vi "PicoScopeospaExampleAdvancedTrigger.vi"() -> ()   [LabVIEW 2010]
uses:
  shared/PicoBuffers.ctl
  <vilib>/Waveform/DWDTOps.llb/DWDT Analog to Digital.vi
  PicoScopepsospaLib/PicoScopeospaDigitalChannelSettings.ctl
  shared/Acquisition Settings.ctl
  shared/Buffer and Transfer Settings.ctl
  PicoScopepsospaLib/PicoScopeospaAnalogChannelSettings.ctl
panel:
  in  "Write ChA to file":bool
  in  "Channels":T1={"Channel A Settings "={"Enabled"=TRUE, "Coupling"=1, "Range"=8, "Analogue Offset"=0.0, "BandWidth"=0, "PROBE_RANGE_INFO"=0}, "Channel B Settings "={"Enabled"=FALSE, "Coupling"=1, "Range"=8, "Analogue Offset"=0.0, "BandWidth"=0, "PROBE_RANGE_INFO"=0}, "Channel C Settings "={"Enabled"=FALSE, "Coupling"=1, "Range"=8, "Analogue Offset"=0.0, "BandWidth"=0, "PROBE_RANGE_INFO"=0}, "Channel D Settings "={"Enabled"=FALSE, "Coupling"=1, "Range"=8, "Analogue Offset"=0.0, "BandWidth"=0, "PROBE_RANGE_INFO"=0}, "Channel E Settings "={"Enabled"=FALSE, "Coupling"=1, "Range"=8, "Analogue Offset"=0.0, "BandWidth"=0, "PROBE_RANGE_INFO"=0}, "Channel F Settings "={"Enabled"=FALSE, "Coupling"=1, "Range"=8, "Analogue Offset"=0.0, "BandWidth"=0, "PROBE_RANGE_INFO"=0}, "Channel G Settings "={"Enabled"=FALSE, "Coupling"=1, "Range"=8, "Analogue Offset"=0.0, "BandWidth"=0, "PROBE_RANGE_INFO"=0}, "Channel H Settings "={"Enabled"=FALSE, "Coupling"=1, "Range"=8, "Analogue Offset"=0.0, "BandWidth"=0, "PROBE_RANGE_INFO"=0}} {"Channel H Settings"."PROBE_RANGE_INFO" items=["PROBE_NONE_NV"=0, "X1_PROBE_NV"=1, "X10_PROBE_NV"=10]; "Channel H Settings"."BandWidth" items=["Full"=0, "100kHz"=100000, "20kHz"=200000, "1MHz"=1000000, "20MHz"=20000000, "25MHz"=25000000, "50MHz"=50000000, "200MHz"=200000000, "250MHz"=250000000, "500MHz"=500000000]; "Channel H Settings"."Range" items=["10mV"=0, "20mV"=1, "50mV"=2, "100mV"=3, "200mV"=4, "500mV"=5, "1V"=6, "2V"=7, "5V"=8, "10V"=9, "20V"=10, "50V"=11, "100V"=12, "200V"=13, "x10_Probe_100mV"=32, "x10_Probe_200mV"=33, "x10_Probe_500mV"=34, "x10_Probe_1V"=35, "x10_Probe_2V"=36, "x10_Probe_5V"=37, "x10_Probe_10V"=38, "x10_Probe_20V"=39, "x10_Probe_50V"=40, "x10_Probe_100V"=41, "x10_Probe_200V"=42, "x10_Probe_500V"=43, "CURRENT_CLAMP_60A_2A"=10500, "CURRENT_CLAMP_60A_5A"=10501, "CURRENT_CLAMP_60A_10A"=10502, "CURRENT_CLAMP_60A_20A"=10503, "CURRENT_CLAMP_60A_50A"=10504, "CURRENT_CLAMP_60A_60A"=10505, "CURRENT_CLAMP_60A_V2_0_5A"=10600, "CURRENT_CLAMP_60A_V2_1A"=10601, "CURRENT_CLAMP_60A_V2_2A"=10602, "CURRENT_CLAMP_60A_V2_5A"=10603, "CURRENT_CLAMP_60A_V2_10A"=10604, "CURRENT_CLAMP_60A_V2_20A"=10605, "CURRENT_CLAMP_60A_V2_50A"=10606, "CURRENT_CLAMP_60A_V2_60A"=10607, "RESISTANCE_LEAD_NEG5_TO_20OHM"=7000, "RESISTANCE_LEAD_NEG50_TO_200OHM"=7001, "RESISTANCE_LEAD_NEG500_TO_2KOHM"=7002, "RESISTANCE_LEAD_NEG5K_TO_20KOHM"=7003, "RESISTANCE_LEAD_NEG50K_TO_LEAD_200KOHM"=7004, "RESISTANCE_LEAD_NEG500K_TO_LEAD_2MOHM"=7005, "RESISTANCE_LEAD_DIODE_TEST"=7006, "HT_NEG3_TO_5KV"=8950, "HT_NEG3_TO_10KV"=8951, "HT_NEG5_TO_20KV"=8952, "HT_NEG5_TO_50KV"=8953, "HT_NEG5_TO_100KV"=8954, "HT_NEG3_TO_5KV_INVERTED"=8955, "HT_NEG3_TO_10KV_INVERTED"=8956, "HT_NEG5_TO_20KV_INVERTED"=8957, "HT_NEG5_TO_50KV_INVERTED"=8958, "HT_NEG5_TO_100KV_INVERTED"=8959, "TEMPERATURE_NEG50_TO_150DEGC"=9000, "PRESSURE_SENSOR_-100k-150k_PASCALS"=9100, "PRESSURE_SENSOR_-100k_TO_400k_PASCALS"=9101, "PRESSURE_SENSOR_-200k_TO_800k_PASCALS"=9102, "PRESSURE_SENSOR_-400k_TO_1600k_PASCALS"=9103, "PRESSURE_SENSOR_-400k_TO_3400k_PASCALS"=9104, "PRESSURE_SENSOR_-150k_TO_1350k_PASCALS"=9105]; "Channel H Settings"."Coupling" items=["AC"=0, "DC 1M Ohm"=1, "DC 50 Ohm"=50]; "Channel G Settings"."PROBE_RANGE_INFO" items=["PROBE_NONE_NV"=0, "X1_PROBE_NV"=1, "X10_PROBE_NV"=10]; "Channel G Settings"."BandWidth" items=["Full"=0, "100kHz"=100000, "20kHz"=200000, "1MHz"=1000000, "20MHz"=20000000, "25MHz"=25000000, "50MHz"=50000000, "200MHz"=200000000, "250MHz"=250000000, "500MHz"=500000000]; "Channel G Settings"."Range" items=["10mV"=0, "20mV"=1, "50mV"=2, "100mV"=3, "200mV"=4, "500mV"=5, "1V"=6, "2V"=7, "5V"=8, "10V"=9, "20V"=10, "50V"=11, "100V"=12, "200V"=13, "x10_Probe_100mV"=32, "x10_Probe_200mV"=33, "x10_Probe_500mV"=34, "x10_Probe_1V"=35, "x10_Probe_2V"=36, "x10_Probe_5V"=37, "x10_Probe_10V"=38, "x10_Probe_20V"=39, "x10_Probe_50V"=40, "x10_Probe_100V"=41, "x10_Probe_200V"=42, "x10_Probe_500V"=43, "CURRENT_CLAMP_60A_2A"=10500, "CURRENT_CLAMP_60A_5A"=10501, "CURRENT_CLAMP_60A_10A"=10502, "CURRENT_CLAMP_60A_20A"=10503, "CURRENT_CLAMP_60A_50A"=10504, "CURRENT_CLAMP_60A_60A"=10505, "CURRENT_CLAMP_60A_V2_0_5A"=10600, "CURRENT_CLAMP_60A_V2_1A"=10601, "CURRENT_CLAMP_60A_V2_2A"=10602, "CURRENT_CLAMP_60A_V2_5A"=10603, "CURRENT_CLAMP_60A_V2_10A"=10604, "CURRENT_CLAMP_60A_V2_20A"=10605, "CURRENT_CLAMP_60A_V2_50A"=10606, "CURRENT_CLAMP_60A_V2_60A"=10607, "RESISTANCE_LEAD_NEG5_TO_20OHM"=7000, "RESISTANCE_LEAD_NEG50_TO_200OHM"=7001, "RESISTANCE_LEAD_NEG500_TO_2KOHM"=7002, "RESISTANCE_LEAD_NEG5K_TO_20KOHM"=7003, "RESISTANCE_LEAD_NEG50K_TO_LEAD_200KOHM"=7004, "RESISTANCE_LEAD_NEG500K_TO_LEAD_2MOHM"=7005, "RESISTANCE_LEAD_DIODE_TEST"=7006, "HT_NEG3_TO_5KV"=8950, "HT_NEG3_TO_10KV"=8951, "HT_NEG5_TO_20KV"=8952, "HT_NEG5_TO_50KV"=8953, "HT_NEG5_TO_100KV"=8954, "HT_NEG3_TO_5KV_INVERTED"=8955, "HT_NEG3_TO_10KV_INVERTED"=8956, "HT_NEG5_TO_20KV_INVERTED"=8957, "HT_NEG5_TO_50KV_INVERTED"=8958, "HT_NEG5_TO_100KV_INVERTED"=8959, "TEMPERATURE_NEG50_TO_150DEGC"=9000, "PRESSURE_SENSOR_-100k-150k_PASCALS"=9100, "PRESSURE_SENSOR_-100k_TO_400k_PASCALS"=9101, "PRESSURE_SENSOR_-200k_TO_800k_PASCALS"=9102, "PRESSURE_SENSOR_-400k_TO_1600k_PASCALS"=9103, "PRESSURE_SENSOR_-400k_TO_3400k_PASCALS"=9104, "PRESSURE_SENSOR_-150k_TO_1350k_PASCALS"=9105]; "Channel G Settings"."Coupling" items=["AC"=0, "DC 1M Ohm"=1, "DC 50 Ohm"=50]; "Channel F Settings"."PROBE_RANGE_INFO" items=["PROBE_NONE_NV"=0, "X1_PROBE_NV"=1, "X10_PROBE_NV"=10]; "Channel F Settings"."BandWidth" items=["Full"=0, "100kHz"=100000, "20kHz"=200000, "1MHz"=1000000, "20MHz"=20000000, "25MHz"=25000000, "50MHz"=50000000, "200MHz"=200000000, "250MHz"=250000000, "500MHz"=500000000]; "Channel F Settings"."Range" items=["10mV"=0, "20mV"=1, "50mV"=2, "100mV"=3, "200mV"=4, "500mV"=5, "1V"=6, "2V"=7, "5V"=8, "10V"=9, "20V"=10, "50V"=11, "100V"=12, "200V"=13, "x10_Probe_100mV"=32, "x10_Probe_200mV"=33, "x10_Probe_500mV"=34, "x10_Probe_1V"=35, "x10_Probe_2V"=36, "x10_Probe_5V"=37, "x10_Probe_10V"=38, "x10_Probe_20V"=39, "x10_Probe_50V"=40, "x10_Probe_100V"=41, "x10_Probe_200V"=42, "x10_Probe_500V"=43, "CURRENT_CLAMP_60A_2A"=10500, "CURRENT_CLAMP_60A_5A"=10501, "CURRENT_CLAMP_60A_10A"=10502, "CURRENT_CLAMP_60A_20A"=10503, "CURRENT_CLAMP_60A_50A"=10504, "CURRENT_CLAMP_60A_60A"=10505, "CURRENT_CLAMP_60A_V2_0_5A"=10600, "CURRENT_CLAMP_60A_V2_1A"=10601, "CURRENT_CLAMP_60A_V2_2A"=10602, "CURRENT_CLAMP_60A_V2_5A"=10603, "CURRENT_CLAMP_60A_V2_10A"=10604, "CURRENT_CLAMP_60A_V2_20A"=10605, "CURRENT_CLAMP_60A_V2_50A"=10606, "CURRENT_CLAMP_60A_V2_60A"=10607, "RESISTANCE_LEAD_NEG5_TO_20OHM"=7000, "RESISTANCE_LEAD_NEG50_TO_200OHM"=7001, "RESISTANCE_LEAD_NEG500_TO_2KOHM"=7002, "RESISTANCE_LEAD_NEG5K_TO_20KOHM"=7003, "RESISTANCE_LEAD_NEG50K_TO_LEAD_200KOHM"=7004, "RESISTANCE_LEAD_NEG500K_TO_LEAD_2MOHM"=7005, "RESISTANCE_LEAD_DIODE_TEST"=7006, "HT_NEG3_TO_5KV"=8950, "HT_NEG3_TO_10KV"=8951, "HT_NEG5_TO_20KV"=8952, "HT_NEG5_TO_50KV"=8953, "HT_NEG5_TO_100KV"=8954, "HT_NEG3_TO_5KV_INVERTED"=8955, "HT_NEG3_TO_10KV_INVERTED"=8956, "HT_NEG5_TO_20KV_INVERTED"=8957, "HT_NEG5_TO_50KV_INVERTED"=8958, "HT_NEG5_TO_100KV_INVERTED"=8959, "TEMPERATURE_NEG50_TO_150DEGC"=9000, "PRESSURE_SENSOR_-100k-150k_PASCALS"=9100, "PRESSURE_SENSOR_-100k_TO_400k_PASCALS"=9101, "PRESSURE_SENSOR_-200k_TO_800k_PASCALS"=9102, "PRESSURE_SENSOR_-400k_TO_1600k_PASCALS"=9103, "PRESSURE_SENSOR_-400k_TO_3400k_PASCALS"=9104, "PRESSURE_SENSOR_-150k_TO_1350k_PASCALS"=9105]; "Channel F Settings"."Coupling" items=["AC"=0, "DC 1M Ohm"=1, "DC 50 Ohm"=50]; "Channel E Settings"."PROBE_RANGE_INFO" items=["PROBE_NONE_NV"=0, "X1_PROBE_NV"=1, "X10_PROBE_NV"=10]; "Channel E Settings"."BandWidth" items=["Full"=0, "100kHz"=100000, "20kHz"=200000, "1MHz"=1000000, "20MHz"=20000000, "25MHz"=25000000, "50MHz"=50000000, "200MHz"=200000000, "250MHz"=250000000, "500MHz"=500000000]; "Channel E Settings"."Range" items=["10mV"=0, "20mV"=1, "50mV"=2, "100mV"=3, "200mV"=4, "500mV"=5, "1V"=6, "2V"=7, "5V"=8, "10V"=9, "20V"=10, "50V"=11, "100V"=12, "200V"=13, "x10_Probe_100mV"=32, "x10_Probe_200mV"=33, "x10_Probe_500mV"=34, "x10_Probe_1V"=35, "x10_Probe_2V"=36, "x10_Probe_5V"=37, "x10_Probe_10V"=38, "x10_Probe_20V"=39, "x10_Probe_50V"=40, "x10_Probe_100V"=41, "x10_Probe_200V"=42, "x10_Probe_500V"=43, "CURRENT_CLAMP_60A_2A"=10500, "CURRENT_CLAMP_60A_5A"=10501, "CURRENT_CLAMP_60A_10A"=10502, "CURRENT_CLAMP_60A_20A"=10503, "CURRENT_CLAMP_60A_50A"=10504, "CURRENT_CLAMP_60A_60A"=10505, "CURRENT_CLAMP_60A_V2_0_5A"=10600, "CURRENT_CLAMP_60A_V2_1A"=10601, "CURRENT_CLAMP_60A_V2_2A"=10602, "CURRENT_CLAMP_60A_V2_5A"=10603, "CURRENT_CLAMP_60A_V2_10A"=10604, "CURRENT_CLAMP_60A_V2_20A"=10605, "CURRENT_CLAMP_60A_V2_50A"=10606, "CURRENT_CLAMP_60A_V2_60A"=10607, "RESISTANCE_LEAD_NEG5_TO_20OHM"=7000, "RESISTANCE_LEAD_NEG50_TO_200OHM"=7001, "RESISTANCE_LEAD_NEG500_TO_2KOHM"=7002, "RESISTANCE_LEAD_NEG5K_TO_20KOHM"=7003, "RESISTANCE_LEAD_NEG50K_TO_LEAD_200KOHM"=7004, "RESISTANCE_LEAD_NEG500K_TO_LEAD_2MOHM"=7005, "RESISTANCE_LEAD_DIODE_TEST"=7006, "HT_NEG3_TO_5KV"=8950, "HT_NEG3_TO_10KV"=8951, "HT_NEG5_TO_20KV"=8952, "HT_NEG5_TO_50KV"=8953, "HT_NEG5_TO_100KV"=8954, "HT_NEG3_TO_5KV_INVERTED"=8955, "HT_NEG3_TO_10KV_INVERTED"=8956, "HT_NEG5_TO_20KV_INVERTED"=8957, "HT_NEG5_TO_50KV_INVERTED"=8958, "HT_NEG5_TO_100KV_INVERTED"=8959, "TEMPERATURE_NEG50_TO_150DEGC"=9000, "PRESSURE_SENSOR_-100k-150k_PASCALS"=9100, "PRESSURE_SENSOR_-100k_TO_400k_PASCALS"=9101, "PRESSURE_SENSOR_-200k_TO_800k_PASCALS"=9102, "PRESSURE_SENSOR_-400k_TO_1600k_PASCALS"=9103, "PRESSURE_SENSOR_-400k_TO_3400k_PASCALS"=9104, "PRESSURE_SENSOR_-150k_TO_1350k_PASCALS"=9105]; "Channel E Settings"."Coupling" items=["AC"=0, "DC 1M Ohm"=1, "DC 50 Ohm"=50]; "Channel D Settings"."BandWidth" items=["Full"=0, "100kHz"=100000, "20kHz"=200000, "1MHz"=1000000, "20MHz"=20000000, "25MHz"=25000000, "50MHz"=50000000, "100MHz"=100000000, "200MHz"=200000000, "250MHz"=250000000, "350MHz"=350000000, "500MHz"=500000000]; "Channel D Settings"."PROBE_RANGE_INFO" items=["PROBE_NONE_NV"=0, "X1_PROBE_NV"=1, "X10_PROBE_NV"=10]; "Channel D Settings"."Range" items=["10mV", "20mV", "50mV", "100mV", "200mV", "500mV", "1V", "2V", "5V", "10V", "20V", "50V", "100V", "200V"]; "Channel D Settings"."Coupling" items=["AC"=0, "DC 1M Ohm"=1, "DC 50 Ohm"=50]; "Channel C Settings"."BandWidth" items=["Full"=0, "100kHz"=100000, "20kHz"=200000, "1MHz"=1000000, "20MHz"=20000000, "25MHz"=25000000, "50MHz"=50000000, "100MHz"=100000000, "200MHz"=200000000, "250MHz"=250000000, "350MHz"=350000000, "500MHz"=500000000]; "Channel C Settings"."PROBE_RANGE_INFO" items=["PROBE_NONE_NV"=0, "X1_PROBE_NV"=1, "X10_PROBE_NV"=10]; "Channel C Settings"."Range" items=["10mV", "20mV", "50mV", "100mV", "200mV", "500mV", "1V", "2V", "5V", "10V", "20V", "50V", "100V", "200V"]; "Channel C Settings"."Coupling" items=["AC"=0, "DC 1M Ohm"=1, "DC 50 Ohm"=50]; "Channel B Settings"."BandWidth" items=["Full"=0, "100kHz"=100000, "20kHz"=200000, "1MHz"=1000000, "20MHz"=20000000, "25MHz"=25000000, "50MHz"=50000000, "100MHz"=100000000, "200MHz"=200000000, "250MHz"=250000000, "350MHz"=350000000, "500MHz"=500000000]; "Channel B Settings"."PROBE_RANGE_INFO" items=["PROBE_NONE_NV"=0, "X1_PROBE_NV"=1, "X10_PROBE_NV"=10]; "Channel B Settings"."Range" items=["10mV", "20mV", "50mV", "100mV", "200mV", "500mV", "1V", "2V", "5V", "10V", "20V", "50V", "100V", "200V"]; "Channel B Settings"."Coupling" items=["AC"=0, "DC 1M Ohm"=1, "DC 50 Ohm"=50]; "Channel A Settings"."PROBE_RANGE_INFO" items=["PROBE_NONE_NV"=0, "X1_PROBE_NV"=1, "X10_PROBE_NV"=10]; "Channel A Settings"."Range" items=["10mV", "20mV", "50mV", "100mV", "200mV", "500mV", "1V", "2V", "5V", "10V", "20V", "50V", "100V", "200V"]; "Channel A Settings"."BandWidth" items=["Full"=0, "100kHz"=100000, "20kHz"=200000, "1MHz"=1000000, "20MHz"=20000000, "25MHz"=25000000, "50MHz"=50000000, "100MHz"=100000000, "200MHz"=200000000, "250MHz"=250000000, "350MHz"=350000000, "500MHz"=500000000]; "Channel A Settings"."Coupling" items=["AC"=0, "DC 1M Ohm"=1, "DC 50 Ohm"=50]}
  in  "Trigger holdoff (Samples)":u64
  in  "Trigger Delay (samples)":u64
  in  "Auto Trigger (us)":u32=1000000 format="%.4p"
  in  "Pulse Width Qualifier Conditions":T2 {"Port 1" items=["Don't Care", "True", "False"]; "Channel H" items=["Don't Care", "True", "False"]; "Channel G" items=["Don't Care", "True", "False"]; "Channel F" items=["Don't Care", "True", "False"]; "Channel E" items=["Don't Care", "True", "False"]; "Aux" items=["Don't Care", "True", "False"]; "Port 0" items=["Don't Care", "True", "False"]; "Channel D" items=["Don't Care", "True", "False"]; "Channel C" items=["Don't Care", "True", "False"]; "Channel B" items=["Don't Care", "True", "False"]; "Channel A" items=["Don't Care", "True", "False"]; "Condition Logic" items=["AND", "OR", "XOR"]}
  in  "Pulse Width Qualifier Settings":T3 {"Pulse Width Type" items=["None", "Less Than", "Greater Than", "In Range", "Out of Range"]}
  in  "Pulse Width Qualifier Trigger Properties":T4={"Channel A Trigger Properties"={"Threshold Mode"=0, "Available"=TRUE, "Direction"=2}, "Channel B Trigger Properties"={"Threshold Mode"=0, "Available"=FALSE, "Direction"=2}, "Channel C Trigger Properties"={"Threshold Mode"=0, "Available"=FALSE, "Direction"=2}, "Channel D Trigger Properties"={"Threshold Mode"=0, "Available"=FALSE, "Direction"=2}, "Channel E Trigger Properties"={"Threshold Mode"=0, "Available"=FALSE, "Direction"=2}, "Channel F Trigger Properties"={"Threshold Mode"=0, "Available"=FALSE, "Direction"=2}, "Channel G Trigger Properties"={"Threshold Mode"=0, "Available"=FALSE, "Direction"=2}, "Channel H Trigger Properties"={"Threshold Mode"=0, "Available"=FALSE, "Direction"=2}, "Port 0 Trigger Properties"={"Threshold Mode"=0, "Available"=FALSE, "Direction"=2}, "Port 1 Trigger Properties"={"Threshold Mode"=0, "Available"=FALSE, "Direction"=2}} {"Port 1 Trigger Properties"."Direction" items=["Rising"=2, "Falling"=3, "Rising Lower"=7, "Above"=0, "Below"=1, "Rising or Falling"=4, "Falling Lower"=8, "Below Lower"=6, "Above Lower"=5]; "Port 1 Trigger Properties"."Threshold Mode" items=["Level", "Window"]; "Port 0 Trigger Properties"."Direction" items=["Rising"=2, "Falling"=3, "Rising Lower"=7, "Above"=0, "Below"=1, "Rising or Falling"=4, "Falling Lower"=8, "Below Lower"=6, "Above Lower"=5]; "Port 0 Trigger Properties"."Threshold Mode" items=["Level", "Window"]; "Channel H Trigger Properties"."Direction" items=["Rising"=2, "Falling"=3, "Rising Lower"=7, "Above"=0, "Below"=1, "Rising or Falling"=4, "Falling Lower"=8, "Below Lower"=6, "Above Lower"=5]; "Channel H Trigger Properties"."Threshold Mode" items=["Level", "Window"]; "Channel G Trigger Properties"."Direction" items=["Rising"=2, "Falling"=3, "Rising Lower"=7, "Above"=0, "Below"=1, "Rising or Falling"=4, "Falling Lower"=8, "Below Lower"=6, "Above Lower"=5]; "Channel G Trigger Properties"."Threshold Mode" items=["Level", "Window"]; "Channel F Trigger Properties"."Direction" items=["Rising"=2, "Falling"=3, "Rising Lower"=7, "Above"=0, "Below"=1, "Rising or Falling"=4, "Falling Lower"=8, "Below Lower"=6, "Above Lower"=5]; "Channel F Trigger Properties"."Threshold Mode" items=["Level", "Window"]; "Channel E Trigger Properties"."Direction" items=["Rising"=2, "Falling"=3, "Rising Lower"=7, "Above"=0, "Below"=1, "Rising or Falling"=4, "Falling Lower"=8, "Below Lower"=6, "Above Lower"=5]; "Channel E Trigger Properties"."Threshold Mode" items=["Level", "Window"]; "Channel D Trigger Properties"."Direction" items=["Rising"=2, "Falling"=3, "Rising Lower"=7, "Above"=0, "Below"=1, "Rising or Falling"=4, "Falling Lower"=8, "Below Lower"=6, "Above Lower"=5]; "Channel D Trigger Properties"."Threshold Mode" items=["Level", "Window"]; "Channel C Trigger Properties"."Direction" items=["Rising"=2, "Falling"=3, "Rising Lower"=7, "Above"=0, "Below"=1, "Rising or Falling"=4, "Falling Lower"=8, "Below Lower"=6, "Above Lower"=5]; "Channel C Trigger Properties"."Threshold Mode" items=["Level", "Window"]; "Channel B Trigger Properties"."Direction" items=["Rising"=2, "Falling"=3, "Rising Lower"=7, "Above"=0, "Below"=1, "Rising or Falling"=4, "Falling Lower"=8, "Below Lower"=6, "Above Lower"=5]; "Channel B Trigger Properties"."Threshold Mode" items=["Level", "Window"]; "Channel A Trigger Properties"."Direction" items=["Rising"=2, "Falling"=3, "Rising Lower"=7, "Above"=0, "Below"=1, "Rising or Falling"=4, "Falling Lower"=8, "Below Lower"=6, "Above Lower"=5]; "Channel A Trigger Properties"."Threshold Mode" items=["Level", "Window"]}
  in  "Digital Ports":T5 {"Digital Port  1"."Direction Channel 15" items=["Don't Care", "Low", "High", "Rising", "Falling"]; "Digital Port  1"."Direction Channel 14" items=["Don't Care", "Low", "High", "Rising", "Falling"]; "Digital Port  1"."Direction Channel 13" items=["Don't Care", "Low", "High", "Rising", "Falling"]; "Digital Port  1"."Direction Channel 12" items=["Don't Care", "Low", "High", "Rising", "Falling"]; "Digital Port  1"."Direction Channel 11" items=["Don't Care", "Low", "High", "Rising", "Falling"]; "Digital Port  1"."Direction Channel 10" items=["Don't Care", "Low", "High", "Rising", "Falling"]; "Digital Port  1"."Direction Channel 9" items=["Don't Care", "Low", "High", "Rising", "Falling"]; "Digital Port  1"."Direction Channel 8" items=["Don't Care", "Low", "High", "Rising", "Falling"]; "Digital Port  0"."Direction Channel 7" items=["Don't Care", "Low", "High", "Rising", "Falling"]; "Digital Port  0"."Direction Channel 6" items=["Don't Care", "Low", "High", "Rising", "Falling"]; "Digital Port  0"."Direction Channel 5" items=["Don't Care", "Low", "High", "Rising", "Falling"]; "Digital Port  0"."Direction Channel 4" items=["Don't Care", "Low", "High", "Rising", "Falling"]; "Digital Port  0"."Direction Channel 3" items=["Don't Care", "Low", "High", "Rising", "Falling"]; "Digital Port  0"."Direction Channel 2" items=["Don't Care", "Low", "High", "Rising", "Falling"]; "Digital Port  0"."Direction Channel 1" items=["Don't Care", "Low", "High", "Rising", "Falling"]; "Digital Port  0"."Direction Channel 0" items=["Don't Care", "Low", "High", "Rising", "Falling"]}
  in  "Channel Trigger Properties":T6={"Channel A Trigger Properties"={"thresholdUpper"=0, "thresholdUpperHysteresis"=1638, "thresholdLower"=0, "thresholdLowerHysteresis"=1638, "Threshold Mode"=0, "Direction"=2, "Available"=TRUE}, "Channel B Trigger Properties"={"thresholdUpper"=0, "thresholdUpperHysteresis"=1638, "thresholdLower"=0, "thresholdLowerHysteresis"=1638, "Threshold Mode"=0, "Direction"=2, "Available"=FALSE}, "Channel C Trigger Properties"={"thresholdUpper"=0, "thresholdUpperHysteresis"=1638, "thresholdLower"=0, "thresholdLowerHysteresis"=1638, "Threshold Mode"=0, "Direction"=2, "Available"=FALSE}, "Channel D Trigger Properties"={"thresholdUpper"=0, "thresholdUpperHysteresis"=1638, "thresholdLower"=0, "thresholdLowerHysteresis"=1638, "Threshold Mode"=0, "Direction"=2, "Available"=FALSE}, "Channel E Trigger Properties"={"thresholdUpper"=0, "thresholdUpperHysteresis"=0, "thresholdLower"=0, "thresholdLowerHysteresis"=0, "Threshold Mode"=0, "Direction"=2, "Available"=FALSE}, "Channel F Trigger Properties"={"thresholdUpper"=0, "thresholdUpperHysteresis"=0, "thresholdLower"=0, "thresholdLowerHysteresis"=0, "Threshold Mode"=0, "Direction"=2, "Available"=FALSE}, "Channel G Trigger Properties"={"thresholdUpper"=0, "thresholdUpperHysteresis"=0, "thresholdLower"=0, "thresholdLowerHysteresis"=0, "Threshold Mode"=0, "Direction"=2, "Available"=FALSE}, "Channel H Trigger Properties"={"thresholdUpper"=0, "thresholdUpperHysteresis"=0, "thresholdLower"=0, "thresholdLowerHysteresis"=0, "Threshold Mode"=0, "Direction"=2, "Available"=FALSE}} {"Channel H Trigger Properties"."Direction" items=["Above / Inside", "Below / Outside", "Rising / Enter", "Falling / Exit", "Rising or Falling / Enter or Exit", "Above Lower", "Below Lower", "Rising Lower", "Falling Lower", "Positive Runt", "Negative Runt"]; "Channel H Trigger Properties"."Threshold Mode" items=["Level", "Window"]; "Channel G Trigger Properties"."Direction" items=["Above / Inside", "Below / Outside", "Rising / Enter", "Falling / Exit", "Rising or Falling / Enter or Exit", "Above Lower", "Below Lower", "Rising Lower", "Falling Lower", "Positive Runt", "Negative Runt"]; "Channel G Trigger Properties"."Threshold Mode" items=["Level", "Window"]; "Channel F Trigger Properties"."Direction" items=["Above / Inside", "Below / Outside", "Rising / Enter", "Falling / Exit", "Rising or Falling / Enter or Exit", "Above Lower", "Below Lower", "Rising Lower", "Falling Lower", "Positive Runt", "Negative Runt"]; "Channel F Trigger Properties"."Threshold Mode" items=["Level", "Window"]; "Channel E Trigger Properties"."Direction" items=["Above / Inside", "Below / Outside", "Rising / Enter", "Falling / Exit", "Rising or Falling / Enter or Exit", "Above Lower", "Below Lower", "Rising Lower", "Falling Lower", "Positive Runt", "Negative Runt"]; "Channel E Trigger Properties"."Threshold Mode" items=["Level", "Window"]; "Channel D Trigger Properties"."Direction" items=["Above / Inside", "Below / Outside", "Rising / Enter", "Falling / Exit", "Rising or Falling / Enter or Exit", "Above Lower", "Below Lower", "Rising Lower", "Falling Lower", "Positive Runt", "Negative Runt"]; "Channel D Trigger Properties"."Threshold Mode" items=["Level", "Window"]; "Channel C Trigger Properties"."Direction" items=["Above / Inside", "Below / Outside", "Rising / Enter", "Falling / Exit", "Rising or Falling / Enter or Exit", "Above Lower", "Below Lower", "Rising Lower", "Falling Lower", "Positive Runt", "Negative Runt"]; "Channel C Trigger Properties"."Threshold Mode" items=["Level", "Window"]; "Channel B Trigger Properties"."Direction" items=["Above / Inside", "Below / Outside", "Rising / Enter", "Falling / Exit", "Rising or Falling / Enter or Exit", "Above Lower", "Below Lower", "Rising Lower", "Falling Lower", "Positive Runt", "Negative Runt"]; "Channel B Trigger Properties"."Threshold Mode" items=["Level", "Window"]; "Channel A Trigger Properties"."Direction" items=["Above / Inside", "Below / Outside", "Rising / Enter", "Falling / Exit", "Rising or Falling / Enter or Exit", "Above Lower", "Below Lower", "Rising Lower", "Falling Lower", "Positive Runt", "Negative Runt"]; "Channel A Trigger Properties"."Threshold Mode" items=["Level", "Window"]}
  in  "Trigger Conditions":T7={"Channel A"=1, "Channel B"=0, "Channel C"=0, "Channel D"=0, "Channel E"=0, "Channel F"=0, "Channel G"=0, "Channel H"=0, "Port 0"=0, "Port 1"=0, "Aux"=0, "PWQ"=0, "Condition Logic"=0} {"Port 1" items=["Don't Care", "True", "False"]; "Channel H" items=["Don't Care", "True", "False"]; "Channel G" items=["Don't Care", "True", "False"]; "Channel F" items=["Don't Care", "True", "False"]; "Channel E" items=["Don't Care", "True", "False"]; "PWQ" items=["Don't Care", "True", "False"]; "Aux" items=["Don't Care", "True", "False"]; "Port 0" items=["Don't Care", "True", "False"]; "Channel D" items=["Don't Care", "True", "False"]; "Channel C" items=["Don't Care", "True", "False"]; "Channel B" items=["Don't Care", "True", "False"]; "Channel A" items=["Don't Care", "True", "False"]; "Condition Logic" items=["AND", "OR", "XOR"]}
  out "error out":errorcluster
  in  "Data file":path=path "PicoScopeospaExampleAdvancedTrigger ChA Data"
  out "overflow":i16 format="%010b"
  in  "Apply Settings":bool
  in  "Digital Channels":T8={"Port 0 Settings "={"Enabled"=FALSE, "Hysteresis"=3, "Threshold Level (Volts)"=[1.0, 1.0, 1.0, 1.0, 1.0, 1.0, 1.0, 1.0]}, "Port 1 Settings"={"Enabled"=FALSE, "Hysteresis"=3, "Threshold Level (Volts)"=[1.0, 1.0, 1.0, 1.0, 1.0, 1.0, 1.0, 1.0]}} {"Port 1 Settings"."Threshold Level (Volts)" format="%#_4p"; "Port 1 Settings"."Hysteresis" items=["PICO_VERY_HIGH_400MV", "PICO_HIGH_200MV", "PICO_NORMAL_100MV", "PICO_LOW_50MV"]; "Port 0 Settings"."Threshold Level (Volts)" format="%#_4p"; "Port 0 Settings"."Hysteresis" items=["PICO_VERY_HIGH_400MV", "PICO_HIGH_200MV", "PICO_NORMAL_100MV", "PICO_LOW_50MV"]}
  in  "Buffer and Transfer Settings":T9={"startIndex"=0, "Samples"=10000000, "Down Sample Ratio"=10, "Down-Sample Mode"=2} {"Down-Sample Mode" items=["RAW none"=2147483648, "None"=0, "Aggregate"=1, "Decimate"=2, "Average"=4]; "Down Sample Ratio" step=1; "Samples" format="%_6p"}
  in  "Acquisition Settings":T10={"preTriggerSamples"=0, "postTriggerSamples"=100000000, "timebase"=2} {"postTriggerSamples" format="%_6p"; "preTriggerSamples" format="%_6p"}
  out "Properties Panel":T11 {"Max Total Capture Time Available (sec)" format="%.3p"; "Sample Frequency" format="%.6p"; "Sample Rate" format="%.3p"; "Max Samples Available" format="%_6p"; "Total Capture Time (sec)" format="%.3p"}
  out "Port 0":digitalwaveform(graph)={"t0"=timestamp(0 s since 1904-01-01), "dt"=8e-09, "Y"={"transitions"=[], "data"=[]}}
  in  "stop":bool
  out "Analog Channels":cluster{i32, dbl, "Data":dbl[]}[](graph)
  out "Device Info":T12={"PICO_DRIVER_VERSION"="psospa Windows Driver, 1.0.91.5523", "PICO_USB_VERSION"="3.0", "PICO_HARDWARE_VERSION"="1.0", "PICO_VARIANT_INFO"="3418E", "PICO_BATCH_AND_SERIAL"="10162/0012", "PICO_CAL_DATE"="08Feb24", "PICO_KERNEL_VERSION"="1", "PICO_DIGITAL_HARDWARE_VERSION"="0", "PICO_ANALOGUE_HARDWARE_VERSION"="1.10.6.0", "PICO_FIRMWARE_VERSION_1"="1.3.13.0", "PICO_FIRMWARE_VERSION_2"="1.4.0-161", "PICO_IPP_VERSION"="C:\\Program Files\\Pico Technology\\SDK\\lib\\psospa.dll", "PICO_DRIVER_PATH"="", "PICO_FIRMWARE_VERSION_3"="", "PICO_FRONT_PANEL_FIRMWARE_VERSION"="", "Number of Channels"=4, "MSO"=FALSE}
  out "Pico ospa Units":string
  in  "Resolution":u32(ring)=10 items=["8-bit"=0, "12-bit"=1, "14-bit"=2, "15-bit"=3, "16-bit"=4, "10-bit"=10]
  in  "Serial Number":string
  in  "Use Serial Number":bool
  in  "error in (no error)":errorcluster
  # "D8-D15"
  # "DO-D7"
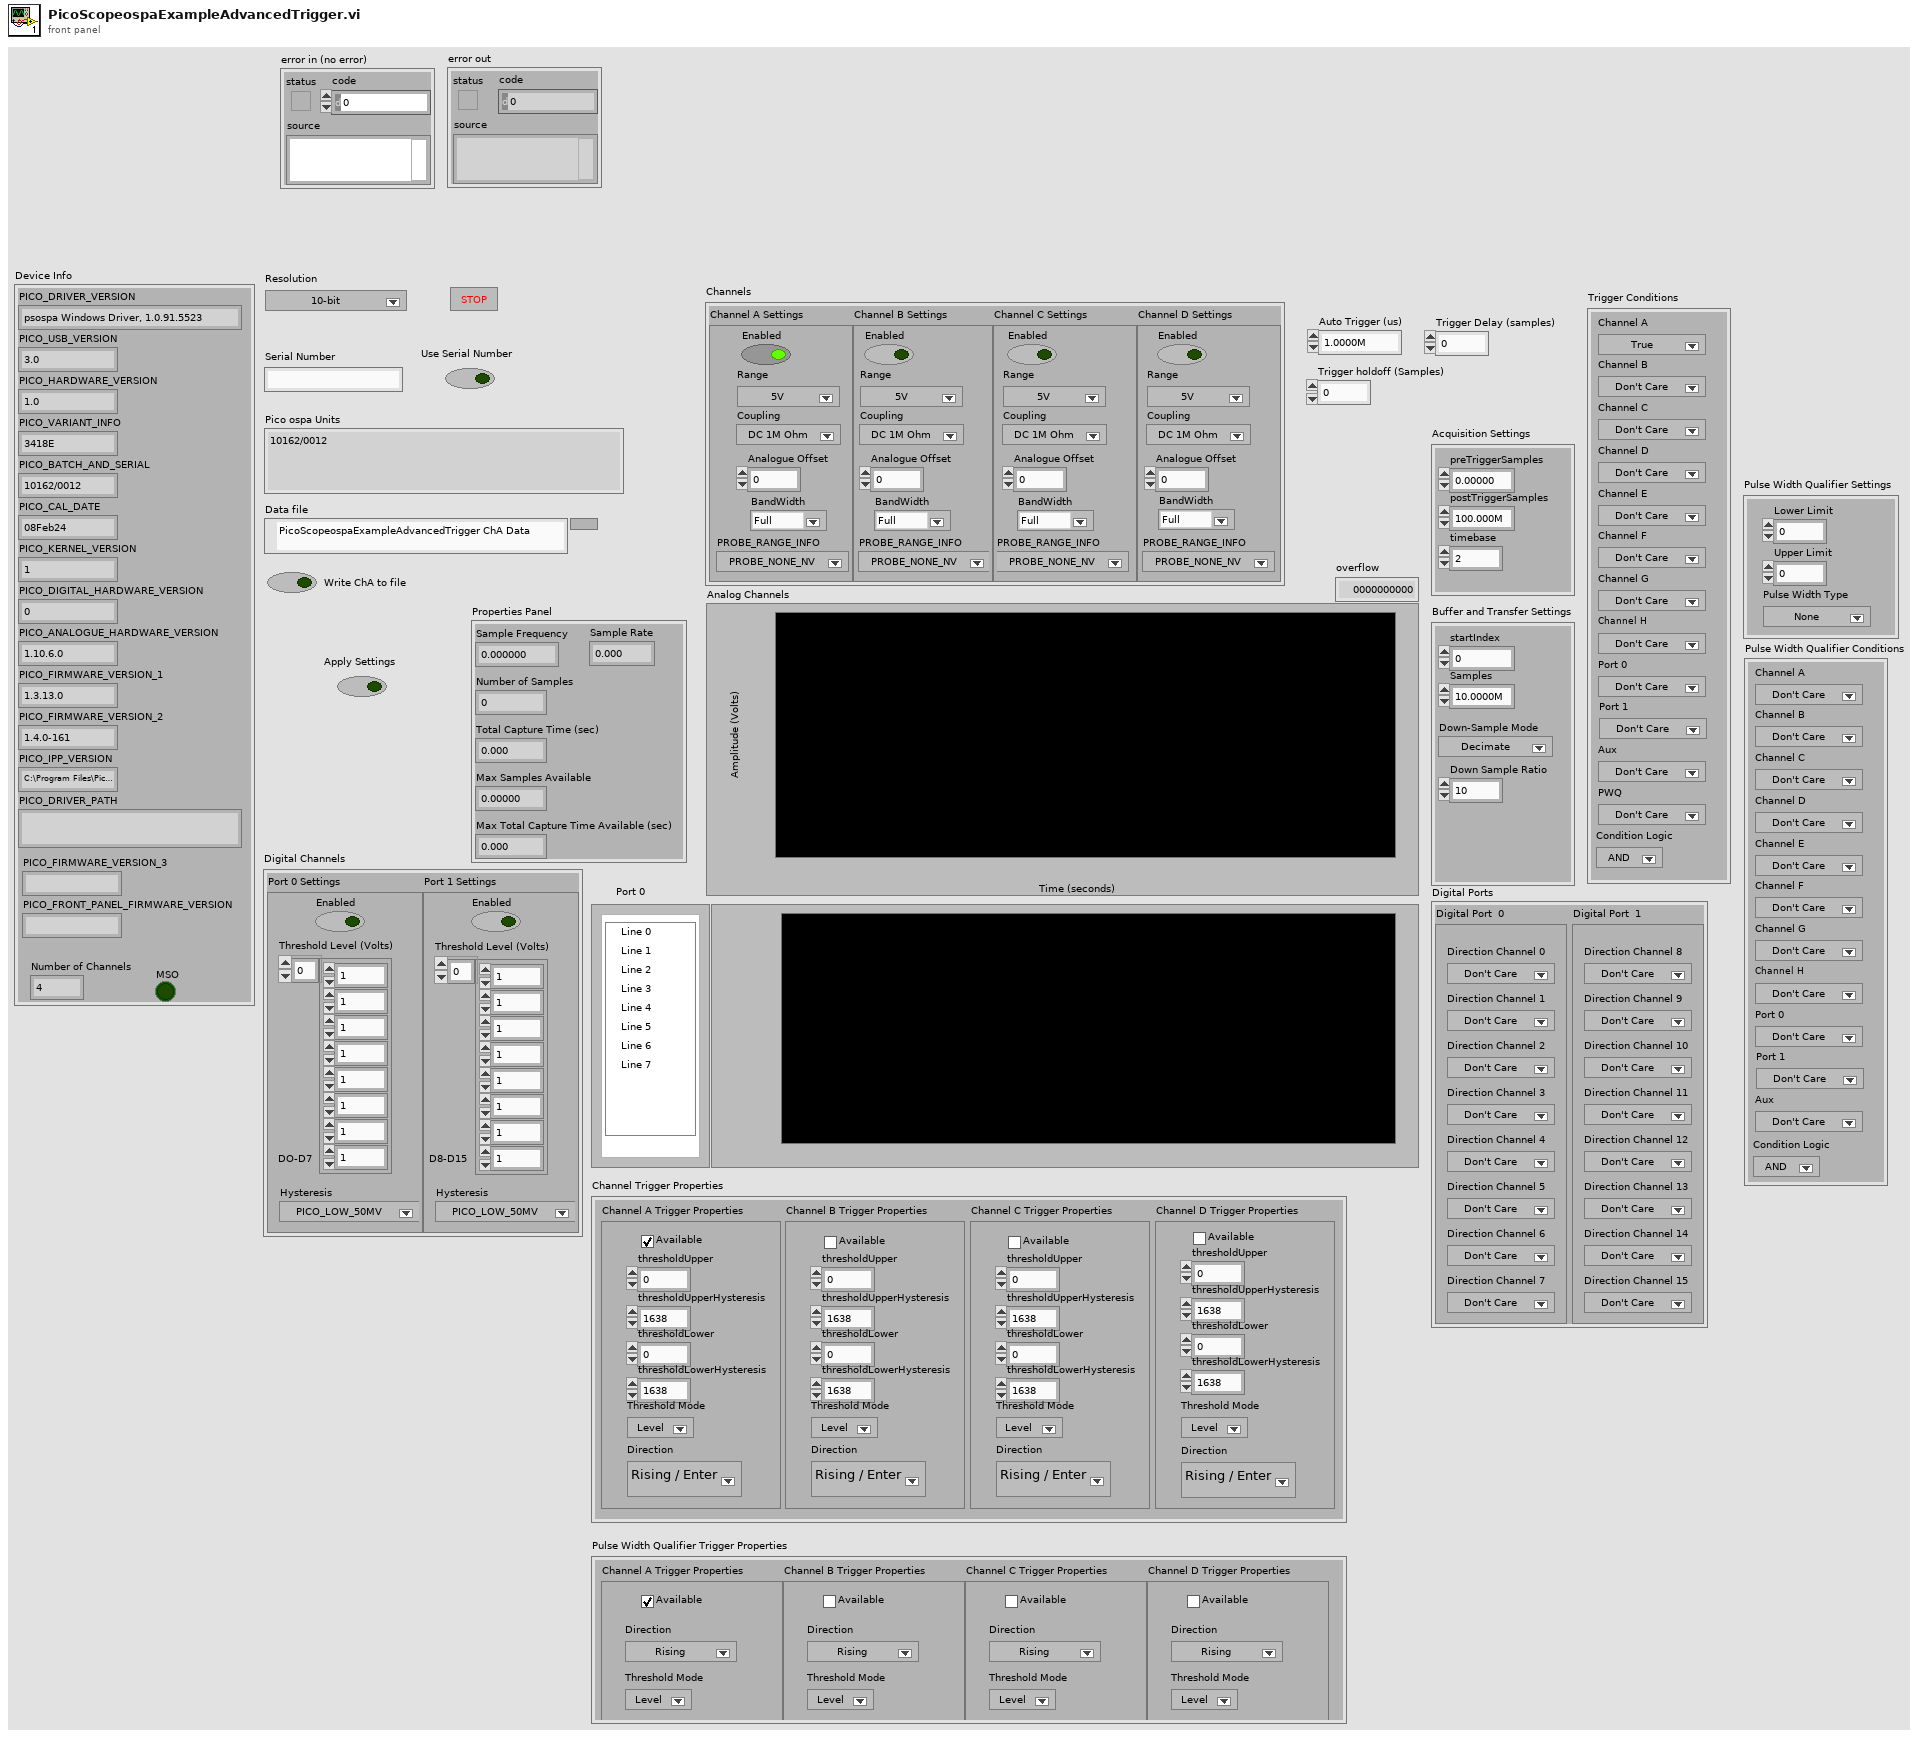
[diagram p1: front panel]
types:
  T1 = typedef "PicoScopeospaAnalogChannelSettings.ctl" = cluster{"Channel A Settings ":cluster{"Enabled":bool, "Coupling":i16, "Range":u16, "Analogue Offset":dbl, "BandWidth":u32, "PROBE_RANGE_INFO":u32}, "Channel B Settings ":cluster{"Enabled":bool, "Coupling":i16, "Range":u16, "Analogue Offset":dbl, "BandWidth":u32, "PROBE_RANGE_INFO":u32}, "Channel C Settings ":cluster{"Enabled":bool, "Coupling":i16, "Range":u16, "Analogue Offset":dbl, "BandWidth":u32, "PROBE_RANGE_INFO":u32}, "Channel D Settings ":cluster{"Enabled":bool, "Coupling":i16, "Range":u16, "Analogue Offset":dbl, "BandWidth":u32, "PROBE_RANGE_INFO":u32}, "Channel E Settings ":cluster{"Enabled":bool, "Coupling":i16, "Range":u16, "Analogue Offset":dbl, "BandWidth":u32, "PROBE_RANGE_INFO":u32}, "Channel F Settings ":cluster{"Enabled":bool, "Coupling":i16, "Range":u16, "Analogue Offset":dbl, "BandWidth":u32, "PROBE_RANGE_INFO":u32}, "Channel G Settings ":cluster{"Enabled":bool, "Coupling":i16, "Range":u16, "Analogue Offset":dbl, "BandWidth":u32, "PROBE_RANGE_INFO":u32}, "Channel H Settings ":cluster{"Enabled":bool, "Coupling":i16, "Range":u16, "Analogue Offset":dbl, "BandWidth":u32, "PROBE_RANGE_INFO":u32}}
  T2 = cluster{"Channel A":u16, "Channel B":u16, "Channel C":u16, "Channel D":u16, "Channel E":u16, "Channel F":u16, "Channel G":u16, "Channel H":u16, "Port 0":u16, "Port 1":u16, "Aux":u16, "Condition Logic":u16}
  T3 = cluster{"Lower Limit":u32, "Upper Limit":u32, "Pulse Width Type":u32}
  T4 = cluster{"Channel A Trigger Properties":cluster{"Threshold Mode":i32, "Available":bool, "Direction":u32}, "Channel B Trigger Properties":cluster{"Threshold Mode":i32, "Available":bool, "Direction":u32}, "Channel C Trigger Properties":cluster{"Threshold Mode":i32, "Available":bool, "Direction":u32}, "Channel D Trigger Properties":cluster{"Threshold Mode":i32, "Available":bool, "Direction":u32}, "Channel E Trigger Properties":cluster{"Threshold Mode":i32, "Available":bool, "Direction":u32}, "Channel F Trigger Properties":cluster{"Threshold Mode":i32, "Available":bool, "Direction":u32}, "Channel G Trigger Properties":cluster{"Threshold Mode":i32, "Available":bool, "Direction":u32}, "Channel H Trigger Properties":cluster{"Threshold Mode":i32, "Available":bool, "Direction":u32}, "Port 0 Trigger Properties":cluster{"Threshold Mode":i32, "Available":bool, "Direction":u32}, "Port 1 Trigger Properties":cluster{"Threshold Mode":i32, "Available":bool, "Direction":u32}}
  T5 = cluster{"Digital Port  0":cluster{"Direction Channel 0":u16, "Direction Channel 1":u16, "Direction Channel 2":u16, "Direction Channel 3":u16, "Direction Channel 4":u16, "Direction Channel 5":u16, "Direction Channel 6":u16, "Direction Channel 7":u16}, "Digital Port  1":cluster{"Direction Channel 8":u16, "Direction Channel 9":u16, "Direction Channel 10":u16, "Direction Channel 11":u16, "Direction Channel 12":u16, "Direction Channel 13":u16, "Direction Channel 14":u16, "Direction Channel 15":u16}}
  T6 = cluster{"Channel A Trigger Properties":cluster{"thresholdUpper":i16, "thresholdUpperHysteresis":u16, "thresholdLower":i16, "thresholdLowerHysteresis":u16, "Threshold Mode":i32, "Direction":i32, "Available":bool}, "Channel B Trigger Properties":cluster{"thresholdUpper":i16, "thresholdUpperHysteresis":u16, "thresholdLower":i16, "thresholdLowerHysteresis":u16, "Threshold Mode":i32, "Direction":i32, "Available":bool}, "Channel C Trigger Properties":cluster{"thresholdUpper":i16, "thresholdUpperHysteresis":u16, "thresholdLower":i16, "thresholdLowerHysteresis":u16, "Threshold Mode":i32, "Direction":i32, "Available":bool}, "Channel D Trigger Properties":cluster{"thresholdUpper":i16, "thresholdUpperHysteresis":u16, "thresholdLower":i16, "thresholdLowerHysteresis":u16, "Threshold Mode":i32, "Direction":i32, "Available":bool}, "Channel E Trigger Properties":cluster{"thresholdUpper":i16, "thresholdUpperHysteresis":u16, "thresholdLower":i16, "thresholdLowerHysteresis":u16, "Threshold Mode":i32, "Direction":i32, "Available":bool}, "Channel F Trigger Properties":cluster{"thresholdUpper":i16, "thresholdUpperHysteresis":u16, "thresholdLower":i16, "thresholdLowerHysteresis":u16, "Threshold Mode":i32, "Direction":i32, "Available":bool}, "Channel G Trigger Properties":cluster{"thresholdUpper":i16, "thresholdUpperHysteresis":u16, "thresholdLower":i16, "thresholdLowerHysteresis":u16, "Threshold Mode":i32, "Direction":i32, "Available":bool}, "Channel H Trigger Properties":cluster{"thresholdUpper":i16, "thresholdUpperHysteresis":u16, "thresholdLower":i16, "thresholdLowerHysteresis":u16, "Threshold Mode":i32, "Direction":i32, "Available":bool}}
  T7 = cluster{"Channel A":u16, "Channel B":u16, "Channel C":u16, "Channel D":u16, "Channel E":u16, "Channel F":u16, "Channel G":u16, "Channel H":u16, "Port 0":u16, "Port 1":u16, "Aux":u16, "PWQ":u16, "Condition Logic":u16}
  T8 = typedef "PicoScopeospaDigitalChannelSettings.ctl" = cluster{"Port 0 Settings ":cluster{"Enabled":bool, "Hysteresis":u32, "Threshold Level (Volts)":dbl[]}, "Port 1 Settings":cluster{"Enabled":bool, "Hysteresis":u32, "Threshold Level (Volts)":dbl[]}}
  T9 = typedef "Buffer and Transfer Settings.ctl" = cluster{"startIndex":u64, "Samples":u64, "Down Sample Ratio":u64, "Down-Sample Mode":u32}
  T10 = typedef "Acquisition Settings.ctl" = cluster{"preTriggerSamples":u64, "postTriggerSamples":u64, "timebase":u32}
  T11 = cluster{"Sample Frequency":dbl, "Sample Rate":dbl, "Max Samples Available":u64, "Number of Samples":u64, "Total Capture Time (sec) ":dbl, "Max Total Capture Time Available (sec)":dbl}
  T12 = cluster{"PICO_DRIVER_VERSION":string, "PICO_USB_VERSION":string, "PICO_HARDWARE_VERSION":string, "PICO_VARIANT_INFO":string, "PICO_BATCH_AND_SERIAL":string, "PICO_CAL_DATE":string, "PICO_KERNEL_VERSION":string, "PICO_DIGITAL_HARDWARE_VERSION":string, "PICO_ANALOGUE_HARDWARE_VERSION":string, "PICO_FIRMWARE_VERSION_1":string, "PICO_FIRMWARE_VERSION_2":string, "PICO_IPP_VERSION":string, "PICO_DRIVER_PATH":string, "PICO_FIRMWARE_VERSION_3":string, "PICO_FRONT_PANEL_FIRMWARE_VERSION":string, "Number of Channels":i16, "MSO":bool}
  T13 = enum16{"open", "open or create", "create or replace", "create", "open (read-only)"}
  T14 = typedef "PicoBuffers.ctl" = cluster{"Max Buffer Pointers":u64[][][], "Min Buffer Pointers":u64[][][], "StreamingDataInfo":cluster{"Channel":u32, "Down-Sample Mode":u32, "PICO_DATA_TYPE":enum32{"PICO_INT8_T", "PICO_INT16_T", "PICO_INT32_T", "PICO_UINT32_T", "PICO_INT64_T", ""}, "Samples":i32, "bufferIndex":u64, "startIndex":i32, "overflow":i16}[][]}
  T15 = cluster{"Channel A Buffer":i16[], "Channel B Buffer":i16[], "Channel C Buffer":i16[], "Channel D Buffer":i16[], "Channel E Buffer":i16[], "Channel F Buffer":i16[], "Channel G Buffer":i16[], "Channel H Buffer":i16[], "Port 0 Buffer":i16[], "Port 1 Buffer":i16[]}[]
  T16 = cluster{"Channel A Buffer":i16[], "Channel B Buffer":i16[], "Channel C Buffer":i16[], "Channel D Buffer":i16[], "Channel E Buffer":i16[], "Channel F Buffer":i16[], "Channel G Buffer":i16[], "Channel H Buffer":i16[], "Port 0 Buffer":i16[], "Port 1 Buffer":i16[]}
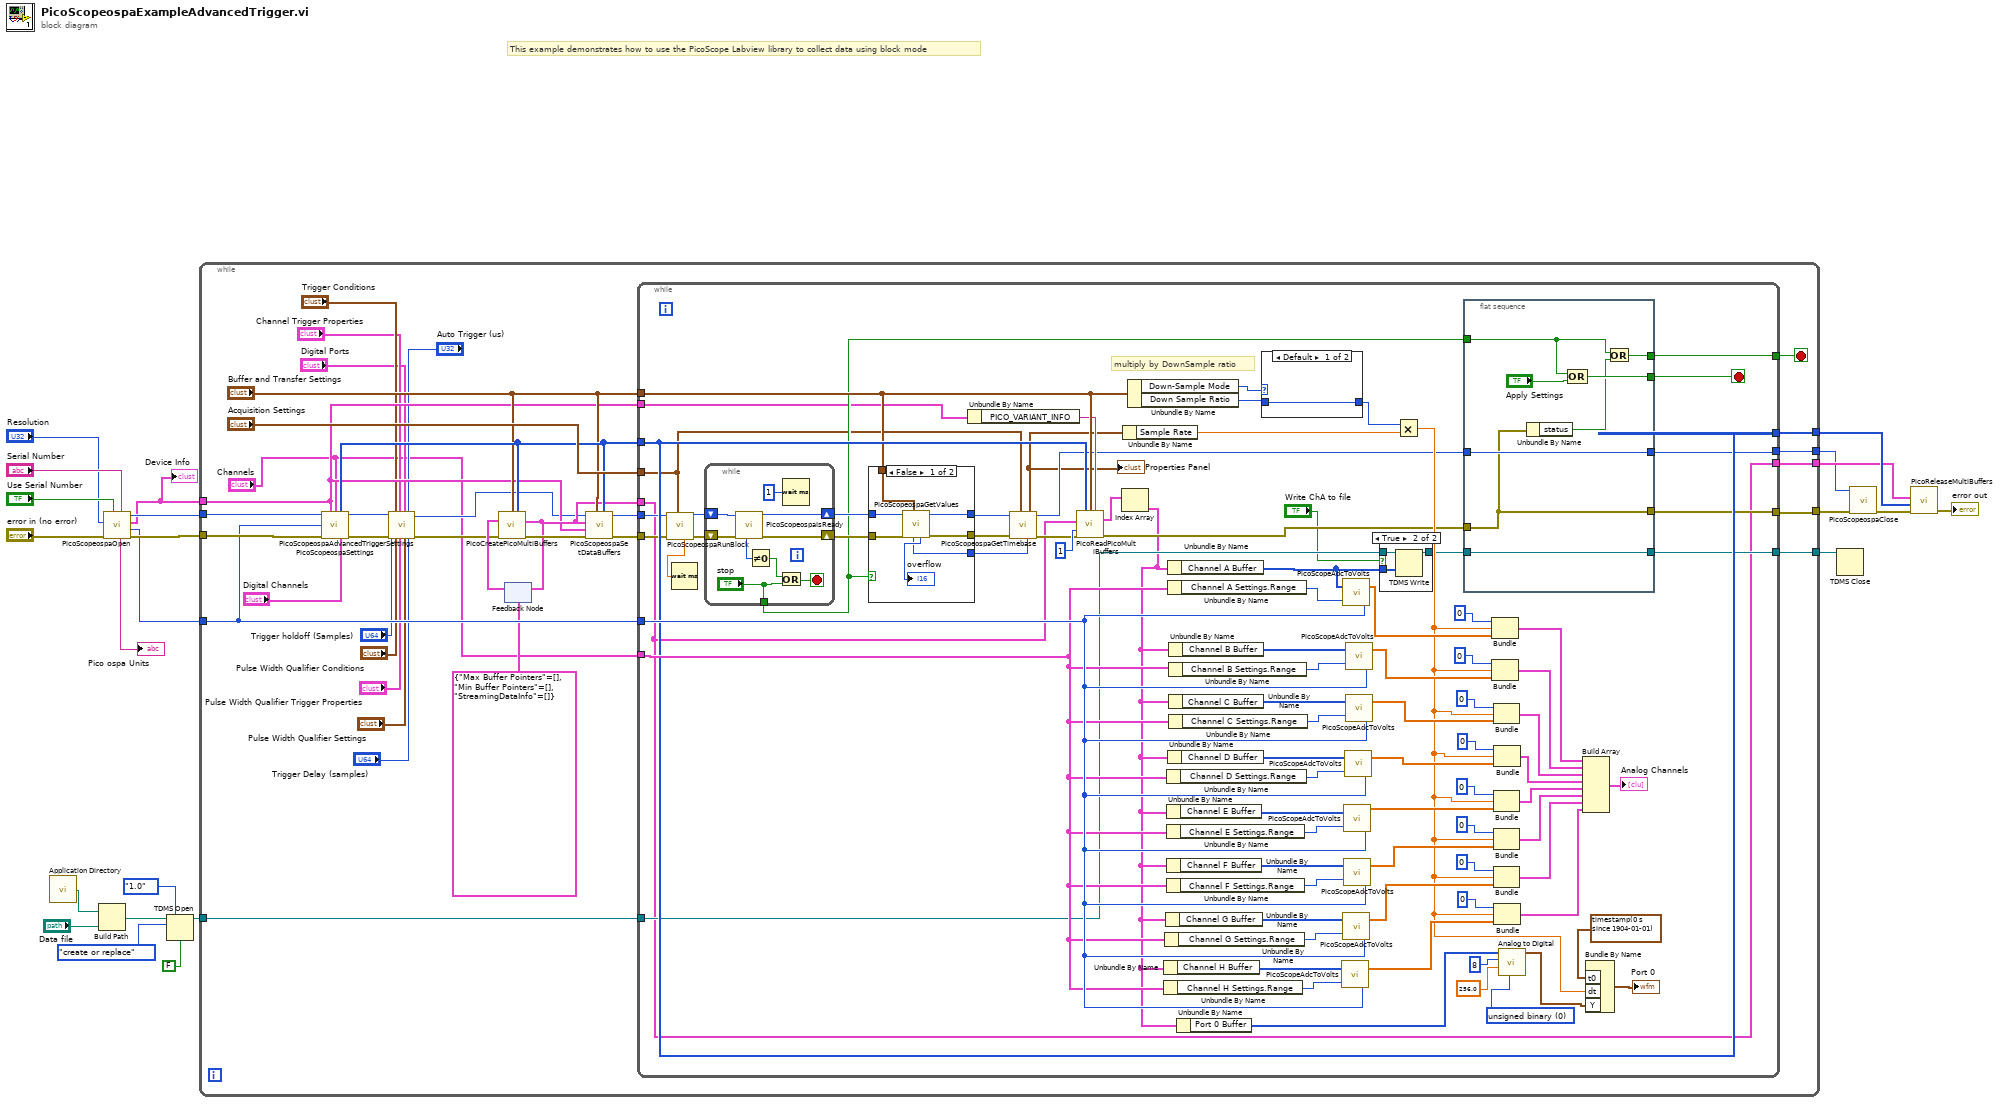
[diagram p0: block diagram]
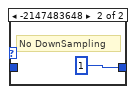
[diagram p4: hidden frame]
diagram:
  # "This example demonstrates how to use the PicoScope Labview library to collect data using block mode"
  n1 = call <vilib>:"Application Directory.vi"() -> ("Application Directory"=w4:path)
  n2 = Build Path(base path=w4, name or relative path="Data file") -> (appended path=w5:path)
  n3 = call "PicoScopeospaOpen.vi"("Serial Number"="Serial Number", "Use Serial Number"="Use Serial Number", "error in (no error)"="error in (no error)", "Resolution"="Resolution") -> ("error out"=w19:errorcluster, "Max ADC value"=w16:i16, "Device Info"=w15:T12, "handle out"=w20:i16, "Pico psospa Units"=→"Pico ospa Units":string)  [unwired: 2 in, 1 out]
  "Device Info" <- w15
  n4 = TDMS Open(6:FALSE ("disable buffering? (T)"), 7:enum16{"1.0", "2.0"}."1.0" ("file format version (2.0)"), 10:T13."create or replace" ("operation (0:open)"), 11:w5) -> (3:w2:refnum<k34>)  [unwired: 2 in, 1 out]
  n5 = while {
    tunnel: w15 -> [w38]
    tunnel: w16 -> [w56]
    tunnel: w20 -> [w58]
    tunnel: [w50] -> w11
    tunnel: w19 -> [w57]
    tunnel: [w49] -> w12
    tunnel: [w48] -> w14
    tunnel: [w52] -> w13
    tunnel: [w40] -> w3
    tunnel: w2 -> [w39]
    stop <- w41 stop-if-true
    n6 = call "PicoScopeospaSettings.vi"("handle in"=w58, "Device Info"=w38, "Channels"="Channels", "Max ADC value"=w56, "error in (no error)"=w57, "Digital Channels"="Digital Channels") -> ("Enabled array"=w45:i16[], "handle out"=w34:i16, "error out"=w37:errorcluster)  [unwired: 7 in]
    n7 = call "PicoScopeospaAdvancedTriggerSettings.vi"("handle in"=w34, "Trigger holdoff (Samples)"="Trigger holdoff (Samples)", "error in"=w37, "Trigger Conditions"="Trigger Conditions", "Pulse Width Qualifier Conditions"="Pulse Width Qualifier Conditions", "Channel Trigger Properties"="Channel Trigger Properties", "Pulse Width Qualifier Trigger Properties"="Pulse Width Qualifier Trigger Properties", "Digital Ports"="Digital Ports", "Pulse Width Qualifier Settings"="Pulse Width Qualifier Settings", "Auto Trigger (us)"="Auto Trigger (us)", "Trigger Delay (samples)"="Trigger Delay (samples)") -> ("handle out"=w35:i16, "error out"=w36:errorcluster)  [unwired: 7 in]
    n8 = feedback #1(T14 {"Max Buffer Pointers"=[], "Min Buffer Pointers"=[], "StreamingDataInfo"=[]} ("Data Pointers")) -> (w51:T14)
    n9 = call "PicoCreatePicoMultiBuffers.vi"("Buffer and Transfer Settings"="Buffer and Transfer Settings", "enabled array"=w45, "Data Pointers In"=w51, "error in (no error)"=w36) -> ("Data Pointers"=w43:T14, "error out"=w47:errorcluster)  [unwired: 10 in]
    n10 = feedback-in #1(w43) -> ()
    n11 = call "PicoScopeospaSetDataBuffers.vi"("enabled array"=w45, "Buffer and Transfer Settings"="Buffer and Transfer Settings", "error in (no error)"=w47, "Device Info"=w38, "Data Pointers In"=w43, "handle in"=w35) -> ("error out"=w46:errorcluster, "handle out"=w42:i16)  [unwired: 4 in]
    n12 = while {
      tunnel: w56 -> [w145]
      tunnel: "Acquisition Settings" -> [w62]
      tunnel: "Channels" -> [w144]
      tunnel: [w78] -> w49
      tunnel: [w61] -> w52
      tunnel: "Buffer and Transfer Settings" -> [w142]
      tunnel: w46 -> [w64]
      tunnel: [w80] -> w50
      tunnel: w42 -> [w63]
      tunnel: w43 -> [w61]
      tunnel: [w143] -> w48
      tunnel: w45 -> [w143]
      tunnel: [w81] -> w41
      tunnel: [w77] -> w40
      tunnel: w39 -> [w75]
      tunnel: w38 -> [w71]
      stop <- w141 stop-if-true
      w101 = u16 0 items=["unsigned binary", "offset binary", "2's complement"] ("data format (offset binary)")
      # "multiply by DownSample ratio"
      n13 = call "PicoScopeospaRunBlock.vi"("Acquisition Settings"=w62, "error in (no error)"=w64, "handle in"=w63) -> ("error out"=w86:errorcluster, "handle out"=w83:i16, "timeIndisposedMs"=w70:dbl)  [unwired: 5 in, 1 out]
      n14 = Wait (ms)(milliseconds to wait=w70) -> ()  [unwired: 1 out]
      n15 = while {
        shift-right: [w174] -> w85
        shift-left: w86 -> [w175]
        shift-right: [w173] -> w84
        shift-left: w83 -> [w172]
        tunnel: ["stop"] -> w82
        stop <- w170 stop-if-true
        n16 = call "PicoScopeospaIsReady.vi"("error in (no error)"=w175, "handle in"=w172) -> ("error out"=w174:errorcluster, "handle out"=w173:i16, "ready"=w171:i16)  [unwired: 7 in]
        n17 = Not Equal To 0?(x=w171) -> (x != 0?=w169:bool)
        n18 = Or(x=w169, y="stop") -> (x .or. y?=w170:bool)
        n19 = Wait (ms)(milliseconds to wait=u32 1) -> ()  [unwired: 1 out]
      }
      n20 = case shown="False" w82 {
        tunnel: w85 -> [w164 w166]
        tunnel: [w163 w166] -> w67
        tunnel: [w162 w165] -> w68
        tunnel: w84 -> [w161 w165]
        tunnel: w142 -> [w160 _]
        tunnel: [w158 _] -> w65
        frame False {
          n21 = call "PicoScopeospaGetValues.vi"("Buffer and Transfer Settings"=w160, "error in (no error)"=w164, "handle in"=w161) -> ("error out"=w163:errorcluster, "handle out"=w162:i16, "overflow"=→"overflow":i16, "noOfSamples"=w158:u64)  [unwired: 5 in]
        }
        frame True {
        }
      }
      n22 = Unbundle By Name(w71) -> ("PICO_VARIANT_INFO"=w72:string)
      n23 = call "PicoScopeospaGetTimebase.vi"("Number of Samples"=w65, "Acquisition Settings"=w62, "error in (no error)"=w67, "handle in"=w68) -> ("error out"=w66:errorcluster, "handle out"=w69:i16, "Properties Panel"=w60:T11)  [unwired: 5 in]
      "Properties Panel" <- w60
      n24 = call "PicoReadPicoMultiBuffers.vi"("enabled array"=w143, "Buffer and Transfer Settings"=w142, "Variant"=w72, "Data Pointers"=w61, "No of Buffers"=1, "error in (no error)"=w66) -> ("MultiBuffers (Max or non-aggregated)"=w93:T15, "error out"=w79:errorcluster)  [unwired: 7 in, 1 out]
      n25 = Index Array(array=w93) -> (element=w74:T16)  [unwired: 1 in]
      n26 = Unbundle By Name(w60) -> ("Sample Rate"=w91:dbl)
      n27 = Unbundle By Name(w142) -> ("Down-Sample Mode"=w89:u32, "Down Sample Ratio"=w90:u64)
      n28 = Unbundle By Name(w74) -> ("Channel H Buffer"=w99:i16[])
      n29 = Unbundle By Name(w144) -> ("Channel H Settings.Range"=w121:u16)
      n30 = Unbundle By Name(w144) -> ("Channel G Settings.Range"=w122:u16)
      n31 = Unbundle By Name(w74) -> ("Channel G Buffer"=w123:i16[])
      n32 = Unbundle By Name(w144) -> ("Channel D Settings.Range"=w128:u16)
      n33 = Unbundle By Name(w74) -> ("Channel E Buffer"=w127:i16[])
      n34 = Unbundle By Name(w144) -> ("Channel E Settings.Range"=w126:u16)
      n35 = Unbundle By Name(w74) -> ("Channel F Buffer"=w125:i16[])
      n36 = Unbundle By Name(w144) -> ("Channel F Settings.Range"=w124:u16)
      n37 = Unbundle By Name(w74) -> ("Channel A Buffer"=w73:i16[])
      n38 = Unbundle By Name(w144) -> ("Channel A Settings.Range"=w139:u16)
      n39 = Unbundle By Name(w74) -> ("Channel D Buffer"=w129:i16[])
      n40 = Unbundle By Name(w74) -> ("Channel B Buffer"=w137:i16[])
      n41 = Unbundle By Name(w144) -> ("Channel B Settings.Range"=w136:u16)
      n42 = Unbundle By Name(w74) -> ("Channel C Buffer"=w131:i16[])
      n43 = Unbundle By Name(w144) -> ("Channel C Settings.Range"=w130:u16)
      n44 = Unbundle By Name(w74) -> ("Port 0 Buffer"=w98:i16[])
      n45 = case shown="Default" w89 {
        tunnel: [w176 u64 1 ("Down Sample Ratio")] -> w87
        tunnel: w90 -> [w176 _]
        frame Default {
        }
        frame -2147483648 {
          # "No DownSampling"
        }
      }
      n46 = call "PicoScopeAdcToVolts.vi"("Max_adc"=w145, "Range Index"=w121, "Data"=w99) -> ("Data"=w116:dbl[])
      n47 = call "PicoScopeAdcToVolts.vi"("Max_adc"=w145, "Range Index"=w139, "Data"=w73) -> ("Data"=w94:dbl[])
      n48 = call "PicoScopeAdcToVolts.vi"("Max_adc"=w145, "Range Index"=w122, "Data"=w123) -> ("Data"=w110:dbl[])
      n49 = call "PicoScopeAdcToVolts.vi"("Max_adc"=w145, "Range Index"=w126, "Data"=w127) -> ("Data"=w113:dbl[])
      n50 = call "PicoScopeAdcToVolts.vi"("Max_adc"=w145, "Range Index"=w124, "Data"=w125) -> ("Data"=w109:dbl[])
      n51 = call "PicoScopeAdcToVolts.vi"("Max_adc"=w145, "Range Index"=w128, "Data"=w129) -> ("Data"=w114:dbl[])
      n52 = call "PicoScopeAdcToVolts.vi"("Max_adc"=w145, "Range Index"=w136, "Data"=w137) -> ("Data"=w135:dbl[])
      n53 = call "PicoScopeAdcToVolts.vi"("Max_adc"=w145, "Range Index"=w130, "Data"=w131) -> ("Data"=w115:dbl[])
      n54 = case shown="True" "Write ChA to file" {
        tunnel: [w146 w149] -> w76
        tunnel: w75 -> [w146 w148]
        tunnel: w73 -> [_ w147]
        frame False {
        }
        frame True {
          n55 = TDMS Write(0:w148, 9:w147) -> (4:w149:refnum<k34>)  [unwired: 4 in, 3 out]
        }
      }
      n56 = Multiply(x=w87, y=w91) -> (x*y=w88:dbl)
      n57 = flat-sequence {
        tunnel: [w157] -> w141
        tunnel: w82 -> [w155]
        tunnel: [w153] -> w81
        tunnel: w69 -> [w152]
        tunnel: [w152] -> w80
        tunnel: w79 -> [w151]
        tunnel: [w151] -> w78
        tunnel: [w150] -> w77
        tunnel: w76 -> [w150]
        frame #0 {
          n58 = Unbundle By Name(w151) -> ("status"=w154:bool)
          n59 = Compound Arithmetic op=OR(w155, "Apply Settings") -> (w157:bool)
          n60 = Or(x=w155, y=w154) -> (x .or. y?=w153:bool)
        }
      }
      n61 = Bundle(0, w88, "Data"=w94) -> (w134:cluster{i32, dbl, "Data":dbl[]})  [unwired: 1 in]
      n62 = Bundle(0, w88, "Data"=w135) -> (w133:cluster{i32, dbl, "Data":dbl[]})  [unwired: 1 in]
      n63 = Bundle(0, w88, "Data"=w115) -> (w108:cluster{i32, dbl, "Data":dbl[]})  [unwired: 1 in]
      n64 = Bundle(0, w88, "Data"=w113) -> (w106:cluster{i32, dbl, "Data":dbl[]})  [unwired: 1 in]
      n65 = Bundle(0, w88, "Data"=w109) -> (w105:cluster{i32, dbl, "Data":dbl[]})  [unwired: 1 in]
      n66 = Bundle(0, w88, "Data"=w110) -> (w104:cluster{i32, dbl, "Data":dbl[]})  [unwired: 1 in]
      n67 = Bundle(0, w88, "Data"=w114) -> (w107:cluster{i32, dbl, "Data":dbl[]})  [unwired: 1 in]
      n68 = Bundle(0, w88, "Data"=w116) -> (w103:cluster{i32, dbl, "Data":dbl[]})  [unwired: 1 in]
      n69 = call-poly <vilib>:"Analog to Digital.vi"("data format (offset binary)"=w101, "full-scale range (pk-pk)"=256.0, "resolution (16 bit)"=8, "analog waveform"=w98) -> ("digital waveform"=w95:digitalwaveform)  [unwired: 4 in, 3 out]
      n70 = Build Array(w134, w133, w108, w107, w106, w105, w104, w103) -> (→"Analog Channels":cluster{i32, dbl, "Data":dbl[]}[])
      n71 = Bundle By Name("t0"=timestamp(0 s since 1904-01-01), "dt"=w88, "Y"=w95) -> (→"Port 0":digitalwaveform)  [unwired: 1 in]
    }
  }
  n72 = TDMS Close(11:w3) -> ()  [unwired: 1 in, 2 out]
  n73 = call "PicoScopeospaClose.vi"("error in (no error)"=w12, "handle in"=w11) -> ("error out"=w10:errorcluster)  [unwired: 8 in, 1 out]
  n74 = call "PicoReleaseMultiBuffers.vi"("error in (no error)"=w10, "Enabled array"=w14, "Data Pointers"=w13) -> ("error out"=→"error out":errorcluster)  [unwired: 7 in, 1 out]
